vi "Send Raw String.vi"(8 "error in (no error)":errorcluster, 10 "Cmd String":string, 11 "Filter Wheel Simulator in":refnum<class "Filter Wheel Simulator.lvclass">) -> (0 "error out":errorcluster, 3 "Filter Wheel Simulator out":refnum<class "Filter Wheel Simulator.lvclass">)   [LabVIEW 2021, in "Filter Wheel Simulator.lvclass"]
uses:
  Filter Wheel Simulator.lvclass
  Filter Wheel Simulator.lvclass/Filter Wheel Simulator.ctl
  Filter Wheel Object/Filter Wheel.lvclass
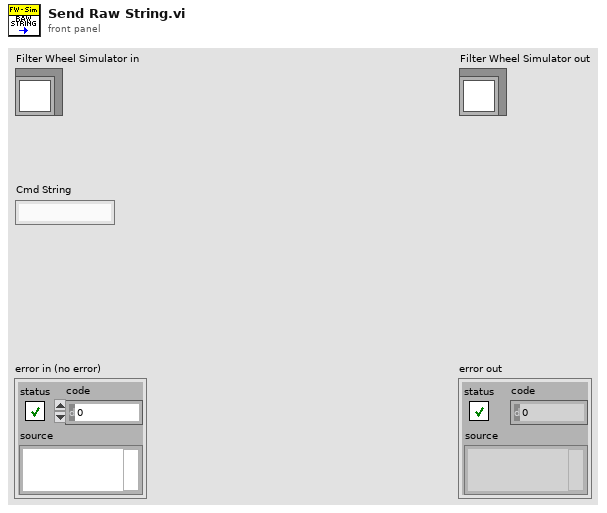
[diagram p1: front panel]
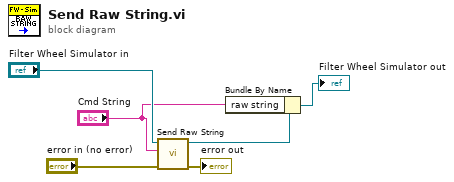
[diagram p0: block diagram]
diagram:
  n1 = call-parent "Send Raw String.vi"("error in (no error)"="error in (no error)", "Cmd String"="Cmd String", "Filter Wheel in"="Filter Wheel Simulator in") -> ("error out"=→"error out":errorcluster, "Filter Wheel out"=w2:refnum<class "Filter Wheel Simulator.lvclass">)  [unwired: 7 in]
  n2 = Bundle By Name(cluster=w2, "raw string"="Cmd String") -> (→"Filter Wheel Simulator out":refnum<class "Filter Wheel Simulator.lvclass">)
